vi "REV2mDistanceSensor Loop.vi"(11 "REV2mDistanceSensorsArray":T1) -> ()   [LabVIEW 2019, in "DistanceSensorDriver.lvlib"]
uses:
  DistanceSensorDriver.lvlib
  Typedef/Rev2mDistanceSensorsArray.ctl
  Typedef/REV2mDistanceSensorDevRef.ctl
  Typedef/Ports.ctl
panel:
  in  "RangeMilliMeter":u16
  in  "RangeStatus":u8
  out "Data Ready":bool
  in  "NewDataReady":u8
  in  "Main Name":string
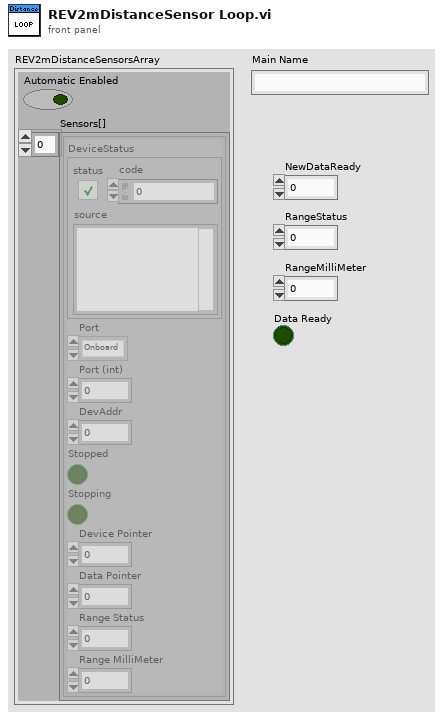
[diagram p1: front panel]
types:
  T1 = typedef "DistanceSensorDriver.lvlib/Rev2mDistanceSensorsArray.ctl" = cluster{"Automatic Enabled":bool, "Sensors[]":T2[]}
  T2 = typedef "DistanceSensorDriver.lvlib/REV2mDistanceSensorDevRef.ctl" = cluster{"DeviceStatus":errorcluster, "Port":T3, "Port (int)":i32, "DevAddr":i32, "Stopped":bool, "Stopping":bool, "Device Pointer":u64, "Data Pointer":u64, "Range Status":u8, "Range MilliMeter":u16}
  T3 = typedef "DistanceSensorDriver.lvlib/Ports.ctl" = enum32{"Onboard", "MXP"}
  T4 = enum32{"Bad", "Idle", "Run top level", "Running"}
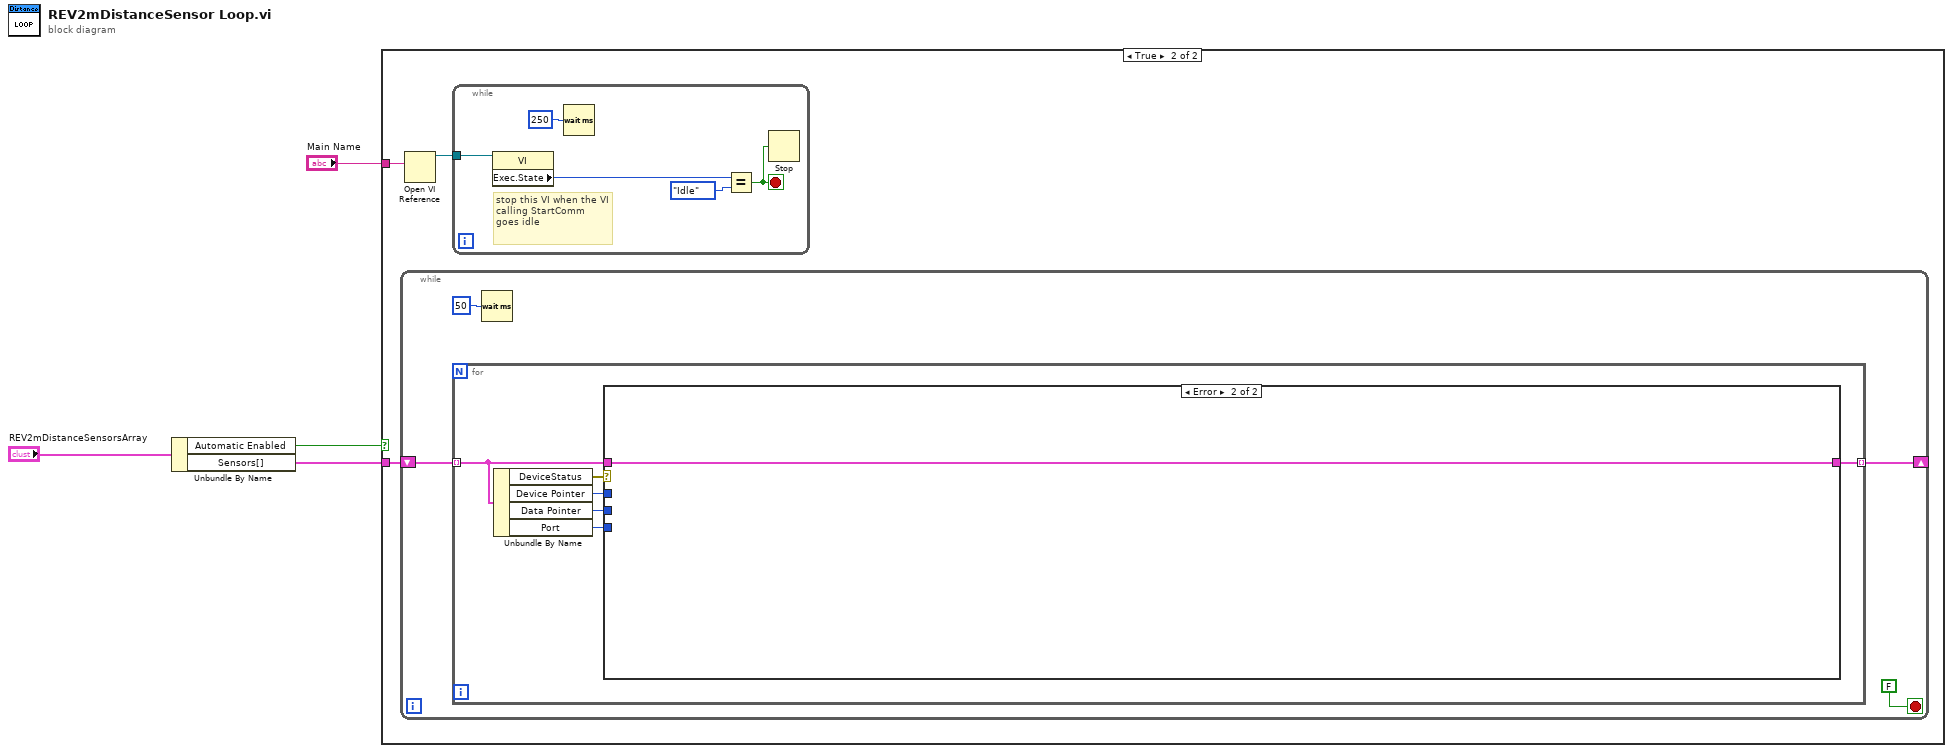
[diagram p0: block diagram]
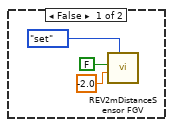
[diagram p2: hidden frame]
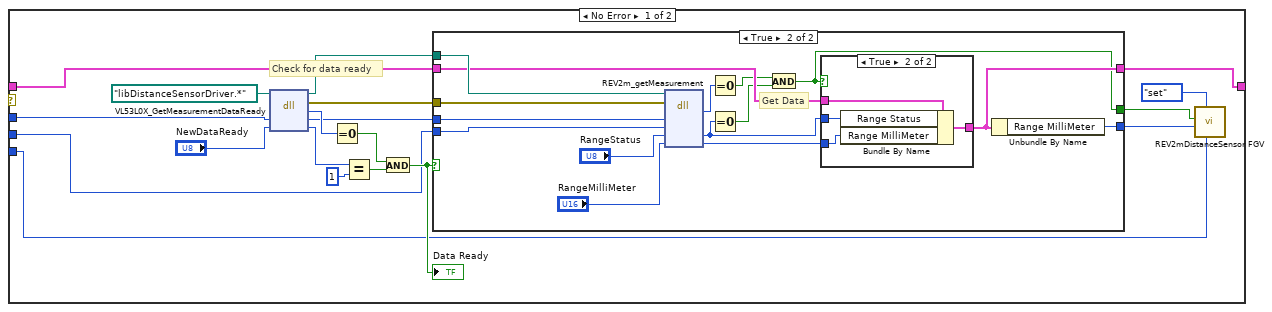
[diagram p3: hidden frame]
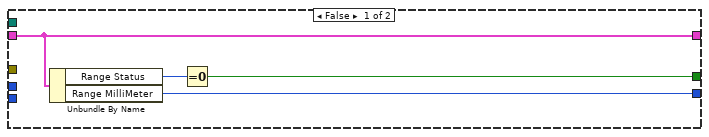
[diagram p4: hidden frame]
diagram:
  n1 = Unbundle By Name("REV2mDistanceSensorsArray") -> ("Automatic Enabled"=w1:bool, "Sensors[]"=w2:T2[])
  n2 = case shown="True" w1 {
    tunnel: "Main Name" -> [_ w9]
    tunnel: w2 -> [_ w8]
    frame False {
      n3 = call "REV2mDistanceSensor FGV.vi"("Operation"=enum16{"set", "get"}."set", "Range"=-2.0 ("Distance"), "Sensor Ready?"=FALSE) -> ()  [unwired: 5 in, 4 out]
    }
    frame True {
      n4 = while {
        shift-right: [w12] -> _
        shift-left: w8 -> [w11]
        stop <- FALSE stop-if-true
        n5 = for {
          tunnel: w11 -> [w18] mode=indexing
          tunnel: [w17] -> w12 mode=indexing
          n6 = Unbundle By Name(w18) -> ("DeviceStatus"=w15:errorcluster, "Device Pointer"=w20:u64, "Data Pointer"=w19:u64, "Port"=w16:T3)
          n7 = case shown="Error" w15 {
            tunnel: w20 -> [w37 _]
            tunnel: w19 -> [w29 _]
            tunnel: w18 -> [w26 w64]
            tunnel: [w25 w64] -> w17
            tunnel: w16 -> [w24 _]
            frame No Error {
              # "Check for data ready"
              n8 = dll-call lib="?" fn="VL53L0X_GetMeasurementDataReady"(path in=path "libDistanceSensorDriver.*", "Dev"=w37, "NewDataReady"="NewDataReady") -> (path out=w28:path, error out=w27:errorcluster, "VL53L0X Error"=w38:i8, "Dev"=w30:u64, "NewDataReady"=w35:u8)  [unwired: 2 in]
              n9 = Equal To 0?(x=w38) -> (x = 0?=w33:bool)
              n10 = Equal?(x=w35, y=u8 1) -> (x = y?=w32:bool)
              n11 = And(x=w33, y=w32) -> (x .and. y?=w31:bool)
              "Data Ready" <- w31
              n12 = case shown="True" w31 {
                tunnel: w30 -> [_ w58]
                tunnel: w29 -> [_ w57]
                tunnel: w28 -> [_ w54]
                tunnel: w27 -> [_ w53]
                tunnel: w26 -> [w43 w51]
                tunnel: [w43 w49] -> w25
                tunnel: [w40 w44] -> w23
                tunnel: [w42 w48] -> w22
                frame False {
                  n13 = Unbundle By Name(w43) -> ("Range Status"=w41:u8, "Range MilliMeter"=w42:u16)
                  n14 = Equal To 0?(x=w41) -> (x = 0?=w40:bool)
                }
                frame True {
                  # "Get Data"
                  n15 = dll-call lib="?" fn="REV2m_getMeasurement"(path in=w54, error in=w53, "pDevice"=w58, "pDat"=w57, "RangeStatus"="RangeStatus", "RangeMilliMeter"="RangeMilliMeter") -> ("VL53L0X Error"=w52:i8, "RangeStatus"=w47:u8, "RangeMilliMeter"=w50:u16)  [unwired: 3 in, 2 out]
                  n16 = Equal To 0?(x=w52) -> (x = 0?=w45:bool)
                  n17 = Equal To 0?(x=w47) -> (x = 0?=w46:bool)
                  n18 = And(x=w45, y=w46) -> (x .and. y?=w44:bool)
                  n19 = case shown="True" w44 {
                    tunnel: w50 -> [_ w62]
                    tunnel: w51 -> [w59 w63]
                    tunnel: [w59 w61] -> w49
                    tunnel: w47 -> [_ w60]
                    frame False {
                    }
                    frame True {
                      n20 = Bundle By Name(cluster=w63, "Range Status"=w60, "Range MilliMeter"=w62) -> (w61:T2)
                    }
                  }
                  n21 = Unbundle By Name(w49) -> ("Range MilliMeter"=w48:u16)
                }
              }
              n22 = call "REV2mDistanceSensor FGV.vi"("Port"=w24, "Operation"=enum16{"set", "get"}."set", "Range"=w22, "Sensor Ready?"=w23) -> ()  [unwired: 4 in, 4 out]
            }
            frame Error {
            }
          }
        }
        n23 = Wait (ms)(milliseconds to wait=u32 50) -> ()  [unwired: 1 out]
      }
      n24 = Open VI Reference(vi path=w9) -> (vi reference=w10:refnum<vi>)  [unwired: 1 in, 5 out]
      n25 = while {
        tunnel: w10 -> [w66]
        stop <- w65 stop-if-true
        # "stop this VI when the VI calling StartComm goes idle"
        n26 = property class="VI"(reference=w66) -> ("Exec.State"=w68:T4)  [unwired: 1 in, 2 out]
        n27 = Wait (ms)(milliseconds to wait=u32 250) -> ()  [unwired: 1 out]
        n28 = Equal?(x=w68, y=T4."Idle" ("Execution:State")) -> (x = y?=w65:bool)
        n29 = Stop(stop? (T)=w65) -> ()
      }
    }
  }
